vi "Rename State Storage.vi"(8 "error in (no error)":errorcluster, 9 "New Name (\"\")":string, 10 "Storage Location (1: 1)":i32(ring)=1 items=["0", "1", "2", "3", "4"], 11 "VISA resource name":refnum<visa-resource-name>) -> (0 "error out":errorcluster, 3 "VISA resource name out":refnum<visa-resource-name>)   [LabVIEW 2016, in "Agilent 3352X Series.lvlib"]
doc: "Assigns a name to the specified storage location.\n\n<b>Note</b>:\n(1) The name will be overwritten when the power is cycled and a new power-down state is stored in this location. \n(2) Deleting the contents of a storage location(Delete State Storage.VI) will reset the associated name to its factory default. \n(3) The factory default names are \"AUTO_RECALL\", \"STATE_1\", \"STATE_2\", \"STATE_3\", and \"STATE_4\"."
uses:
  Agilent 3352X Series.lvlib
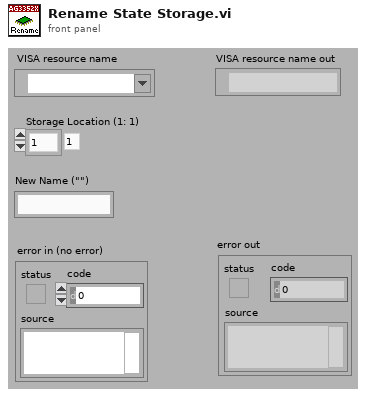
[diagram p1: front panel]
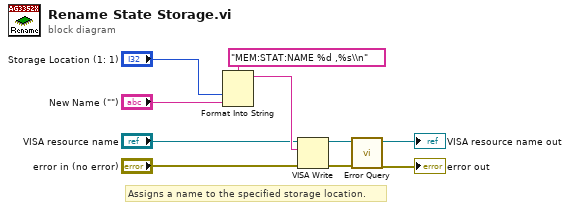
[diagram p0: block diagram]
diagram:
  # "Assigns a name to the specified storage location."
  n1 = Format Into String(format string="MEM:STAT:NAME %d ,%s\\n", "Storage Location (1: 1)", "New Name (\"\")") -> (resulting string=w7:string)  [unwired: 2 in, 1 out]
  n2 = VISA Write(VISA resource name="VISA resource name", write buffer=w7, error in (no error)="error in (no error)") -> (VISA resource name out=w4:refnum<visa-resource-name>, error out=w3:errorcluster)  [unwired: 1 out]
  n3 = call "Error Query.vi"("error in (no error)"=w3, "VISA resource name"=w4) -> ("error out"=→"error out":errorcluster, "VISA resource name out"=→"VISA resource name out":refnum<visa-resource-name>)  [unwired: 8 out]
